vi "ABCtoDQ_noSine_3PhaseUnitaryMagnitude_src.vi"(0 "A":sgl, 1 "cosx":sgl, 2 "sinx":sgl, 5 "B":sgl, 7 "C":sgl) -> (4 "direct":sgl, 6 "quadrature":sgl, 10 "alpha":sgl, 15 "beta":sgl)   [LabVIEW 2015]
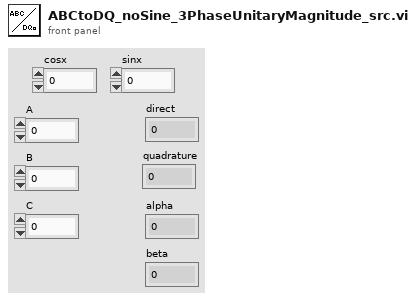
[diagram p1: front panel]
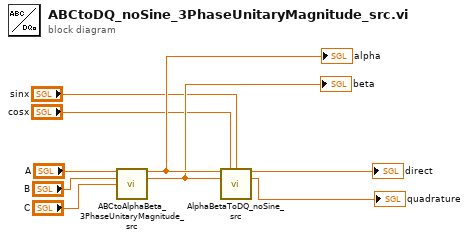
[diagram p0: block diagram]
diagram:
  n1 = call "ABCtoAlphaBeta_3PhaseUnitaryMagnitude_src.vi"("A"="A", "B"="B", "C"="C") -> ("alpha"=w9:sgl, "beta"=w8:sgl)  [unwired: 11 in]
  "alpha" <- w9
  "beta" <- w8
  n2 = call "AlphaBetaToDQ_noSine_src.vi"("alpha"=w9, "cosx"="cosx", "sinx"="sinx", "beta"=w8) -> ("direct"=→"direct":sgl, "quadrature"=→"quadrature":sgl)  [unwired: 10 in]
